vi "Get settings chain.vi"(8 "error in (no error)":errorcluster, 11 "AutofocusBase in":refnum<class "Autofocus.lvclass">) -> (0 "error out":errorcluster, 1 "class name":string[](array[string]), 2 "settings":variant[](array[variant]), 3 "AutofocusBase out":refnum<class "Autofocus.lvclass">)   [LabVIEW 2012, in "Autofocus.lvclass"]
doc: "Returns an array of variants containing the settings clusters of each class in the inheritance chain (lowest child class first), together with an array of all class names in the inheritance chain.\n\nFor classes without settings cluster, the settings chain contains empty variants."
uses:
  Autofocus.lvclass
  <vilib>/Distrio/Murmex/Murmex/Murmex.lvclass
  Autofocus.lvclass/Autofocus.ctl
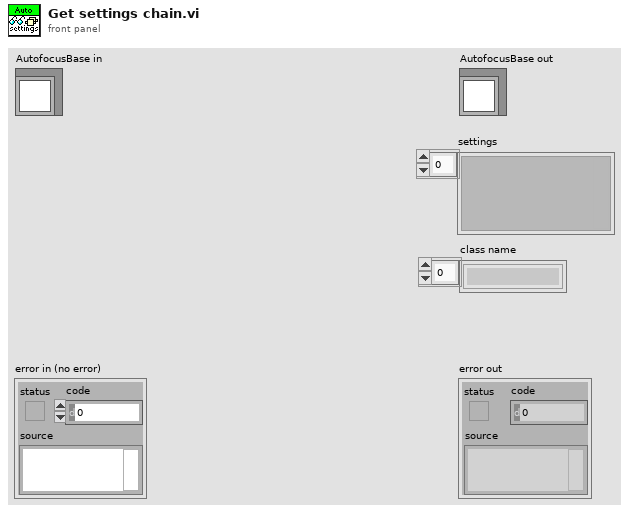
[diagram p1: front panel]
types:
  T1 = typedef "Autofocus.lvclass/settings cluster.ctl" = cluster{"Sharpness measure":T2, "ROI size":T3, "Search Algorithm":T4, "Region sampling":bool, "HC step size":dbl[unit], "current_position_focus":dbl[unit], "threshold":dbl, "brightest percentage":dbl, "number_of_checkpoints":u16, "current_stack_x":dbl[unit], "current_stack_y":dbl[unit], "curent_stack_z1":dbl[unit], "current_stack_z2":dbl[unit], "number_of_stacks":u16, "focus_start":dbl[unit], "focus_stop":dbl[unit], "frames_focus_stack":u16, "Image acquisition mode":T5, "frame rate":dbl[unit]}
  T2 = typedef "Autofocus.lvclass/Sharpness Measure.ctl" = enum16{"Vol4", "Gradient Square"}
  T3 = typedef "Autofocus.lvclass/ROI size.ctl" = u16
  T4 = typedef "Autofocus.lvclass/Search algorithm.ctl" = enum16{"Hill Climbing", "HC+GS"}
  T5 = typedef "Autofocus.lvclass/image acquisition mode.ctl" = enum16{"Focus Stack", "Single Frame"}
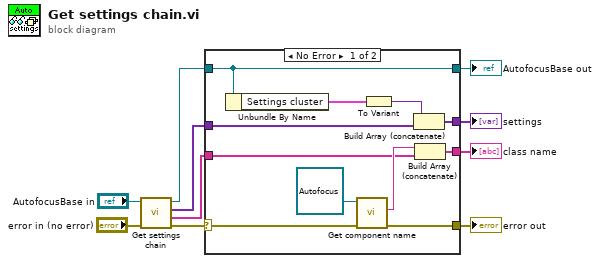
[diagram p0: block diagram]
diagram:
  n1 = call-parent "Get settings chain.vi"("error in (no error)"="error in (no error)", "MurmexBase in"="AutofocusBase in") -> ("error out"=w8:errorcluster, "class name"=w6:string[], "settings"=w1:variant[], "MurmexBase out"=w4:refnum<class "Autofocus.lvclass">)  [unwired: 6 in]
  n2 = case shown="No Error" w8 {
    selector: w8 -> [w21 w23]
    tunnel: [w17 w23] -> w7
    tunnel: w6 -> [w16 _]
    tunnel: [w15 _] -> w5
    tunnel: w4 -> [w14 w22]
    tunnel: [w14 w22] -> w3
    tunnel: [w12 _] -> w2
    tunnel: w1 -> [w11 _]
    frame No Error {
      n3 = Unbundle By Name(w14) -> ("Settings cluster"=w13:T1)
      n4 = call <vilib>:"Get component name.vi"("error in (no error)"=w21, "Murmex in"=refnum<class "Autofocus.lvclass"> refnum ("Autofocus.lvclass")) -> ("error out"=w17:errorcluster, "component name"=w18:string)  [unwired: 7 in, 1 out]
      n5 = To Variant(anything=w13) -> (Variant=w19:variant)
      n6 = Build Array (concatenate)(w19, w11) -> (w12:variant[])
      n7 = Build Array (concatenate)(w18, w16) -> (w15:string[])
    }
    frame Error {
    }
  }
  "error out" <- w7
  "AutofocusBase out" <- w3
  "settings" <- w2
  "class name" <- w5
